vi "byte34-39 (SubVI).vi"(11 "unsigned byte array":u8[](array[numeric])) -> (1 "Numeric 2":u16, 2 "Numeric":u16, 3 "Numeric 3":u16)   [LabVIEW 2016]
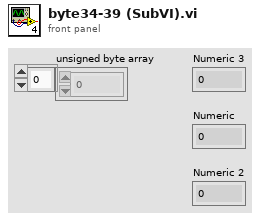
[diagram p1: front panel]
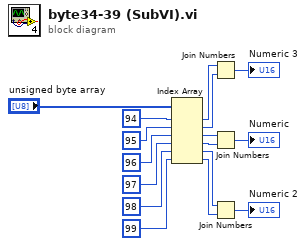
[diagram p0: block diagram]
diagram:
  n1 = Index Array(array="unsigned byte array", index #1=94 ("index"), index #2=95 ("index"), index #3=96 ("index"), index #4=97 ("index"), index #5=98 ("index"), index #6=99 ("index")) -> (element #1=w7:u8, element #2=w8:u8, element #3=w9:u8, element #4=w10:u8, element #5=w11:u8, element #6=w12:u8)
  n2 = Join Numbers(hi=w7, lo=w8) -> ((hi.lo)=→"Numeric 3":u16)
  n3 = Join Numbers(hi=w9, lo=w10) -> ((hi.lo)=→"Numeric":u16)
  n4 = Join Numbers(hi=w11, lo=w12) -> ((hi.lo)=→"Numeric 2":u16)
